vi "Framework Plugin Configuration Test.vi"() -> ()   [LabVIEW 2016]
uses:
  <vilib>/NI Veristand/VeriStand Data/Typedefs/Typedefs.Data Types.ctl
  Classes/Configuration.Transfer/Configuration.Transfer.lvclass
  Classes/Configuration.Channel/Configuration.Channel.lvclass
  Typedefs/Decimation Factors.ctl
  Classes/Plugin Model.UDP/Typedefs/UDP.Transfer Config.ctl
  Classes/Configuration.Transfer Group/Configuration.Transfer Group.lvclass
  Classes/Configuration.Channel/Configuration.Channel.lvclass/Configuration.Channel.ctl
  Classes/Configuration.Transfer/Configuration.Transfer.lvclass/Configuration.Transfer.ctl
  Classes/Configuration.Transfer Group/Configuration.Transfer Group.lvclass/Configuration.Transfer Group.ctl
  Classes/Plugin Model/Plugin Configuration.lvclass/Plugin Configuration.ctl
  Classes/Configuration.Channel/Properties/Write data type.vi
  Classes/Configuration.Channel/Properties/Write offset.vi
  Classes/Configuration.Transfer/Properties/Write byte order.vi
  Classes/Configuration.Transfer/Properties/Write decimation factors.vi
  Classes/Configuration.Transfer/Properties/Write Channels.vi
  Classes/Configuration.Transfer/Properties/Write custom config.vi
  Classes/Configuration.Transfer Group/Properties/Write Transfers.vi
  Classes/Plugin Model/Properties/Write Transfer Groups.vi
  Classes/Plugin Model.UDP/Plugin Configuration.UDP.lvclass
  C:/Users/Ryan/Documents/Git/Sourcetree/VeriStand-Data-Sharing-Framework/Source/Classes/Plugin Model/Plugin Configuration.lvclass
  <vilib>/NI Veristand/VeriStand Data/VeriStand Data.lvlib
  Classes/Plugin Model/Plugin Configuration.lvclass
panel:
  out "resource url":string
  out "Channels":cluster{"offset":u64, "data type":T1}[](array[cluster])
  out "required buffer size in bytes":u64
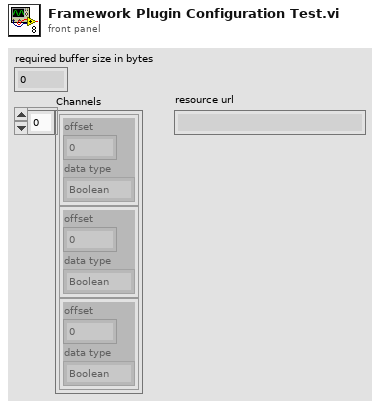
[diagram p1: front panel]
types:
  T1 = typedef "VeriStand Data.lvlib/Typedefs.Data Types.ctl" = enum16{"Boolean", "Single", "Double", "I8", "I16", "I32", "I64", "U8", "U16", "U32", "U64"}
  T2 = typedef "Plugin Configuration.UDP.lvclass/UDP.Transfer Config.ctl" = cluster{"port or service name":u16, "address":u32}
  T3 = typedef "Decimation Factors.ctl" = cluster{"decimation":u16, "offset":u16}
  T4 = enum16{"big-endian, network order", "native, host order", "little-endian"}
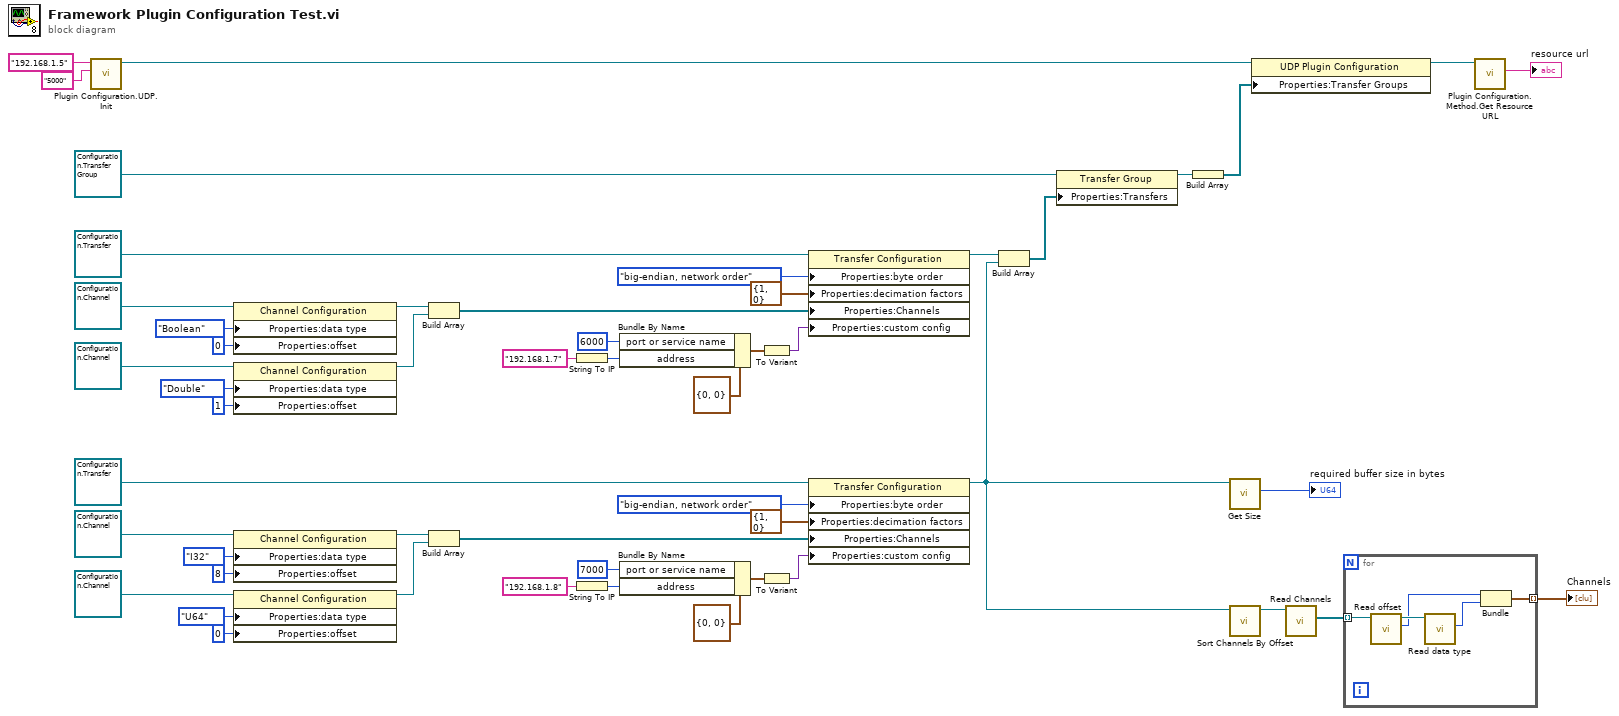
[diagram p0: block diagram]
diagram:
  n1 = call "Plugin Configuration.UDP.Init.vi"("Port"="5000", "IP Address"="192.168.1.5") -> ("UDP Plugin Configuration"=w1:refnum<class "Plugin Configuration.UDP.lvclass">)  [unwired: 8 in, 1 out]
  n2 = property class="Channel Configuration"(reference=refnum<class "Configuration.Channel.lvclass"> refnum ("Channel Configuration"), "Properties:data type"=Typedefs.Data_Types."Boolean" ("data type"), "Properties:offset"=u64 0 ("offset")) -> (reference out=w48:refnum<class "Configuration.Channel.lvclass">)  [unwired: 1 in, 1 out]
  n3 = property class="Channel Configuration"(reference=refnum<class "Configuration.Channel.lvclass"> refnum ("Channel Configuration"), "Properties:data type"=Typedefs.Data_Types."Double" ("data type"), "Properties:offset"=u64 1 ("offset")) -> (reference out=w47:refnum<class "Configuration.Channel.lvclass">)  [unwired: 1 in, 1 out]
  n4 = property class="Channel Configuration"(reference=refnum<class "Configuration.Channel.lvclass"> refnum ("Channel Configuration"), "Properties:data type"=Typedefs.Data_Types."I32" ("data type"), "Properties:offset"=u64 8 ("offset")) -> (reference out=w39:refnum<class "Configuration.Channel.lvclass">)  [unwired: 1 in, 1 out]
  n5 = property class="Channel Configuration"(reference=refnum<class "Configuration.Channel.lvclass"> refnum ("Channel Configuration"), "Properties:data type"=Typedefs.Data_Types."U64" ("data type"), "Properties:offset"=u64 0 ("offset")) -> (reference out=w38:refnum<class "Configuration.Channel.lvclass">)  [unwired: 1 in, 1 out]
  n6 = Build Array(w48, w47) -> (w46:refnum<class "Configuration.Channel.lvclass">[])
  n7 = Build Array(w39, w38) -> (w37:refnum<class "Configuration.Channel.lvclass">[])
  n8 = String To IP(1:"192.168.1.7" ("name")) -> (0:w13:u32)
  n9 = String To IP(1:"192.168.1.8" ("name")) -> (0:w8:u32)
  n10 = Bundle By Name(cluster=T2 {"port or service name"=0, "address"=0} ("UDP transfer config"), "port or service name"=u16 6000, "address"=w13) -> (w17:T2)
  n11 = Bundle By Name(cluster=T2 {"port or service name"=0, "address"=0} ("UDP transfer config"), "port or service name"=u16 7000, "address"=w8) -> (w11:T2)
  n12 = To Variant(anything=w17) -> (Variant=w16:variant)
  n13 = To Variant(anything=w11) -> (Variant=w7:variant)
  n14 = property class="Transfer Configuration"(reference=refnum<class "Configuration.Transfer.lvclass"> refnum ("Transfer Configuration"), "Properties:byte order"=T4."big-endian, network order" ("byte order"), "Properties:decimation factors"=T3 {"decimation"=1, "offset"=0} ("decimation factors"), "Properties:Channels"=w46, "Properties:custom config"=w16) -> (reference out=w34:refnum<class "Configuration.Transfer.lvclass">)  [unwired: 1 in, 1 out]
  n15 = property class="Transfer Configuration"(reference=refnum<class "Configuration.Transfer.lvclass"> refnum ("Transfer Configuration"), "Properties:byte order"=T4."big-endian, network order" ("byte order"), "Properties:decimation factors"=T3 {"decimation"=1, "offset"=0} ("decimation factors"), "Properties:Channels"=w37, "Properties:custom config"=w7) -> (reference out=w22:refnum<class "Configuration.Transfer.lvclass">)  [unwired: 1 in, 1 out]
  n16 = Build Array(w34, w22) -> (w5:refnum<class "Configuration.Transfer.lvclass">[])
  n17 = property class="Transfer Group"(reference=refnum<class "Configuration.Transfer Group.lvclass"> refnum ("Configuration.Transfer Group.lvclass"), "Properties:Transfers"=w5) -> (reference out=w3:refnum<class "Configuration.Transfer Group.lvclass">)  [unwired: 1 in, 1 out]
  n18 = Build Array(w3) -> (w2:refnum<class "Configuration.Transfer Group.lvclass">[])
  n19 = call "Get Size.vi"("Transfer Configuration in"=w22) -> ("size in bytes"=→"required buffer size in bytes":u64)  [unwired: 8 in, 2 out]
  n20 = call "Sort Channels By Offset.vi"("Transfer Configuration in"=w22) -> ("Transfer Configuration out"=w25:refnum<class "Configuration.Transfer.lvclass">)  [unwired: 9 in, 1 out]
  n21 = property class="UDP Plugin Configuration"(reference=w1, "Properties:Transfer Groups"=w2) -> (reference out=w20:refnum<class "Plugin Configuration.UDP.lvclass">)  [unwired: 1 in, 1 out]
  n22 = call "Read Channels.vi"("Configuration.Transfer in"=w25) -> ("Channels"=w24:refnum<class "Configuration.Channel.lvclass">[])  [unwired: 8 in, 2 out]
  n23 = for {
    tunnel: w24 -> [w56] mode=indexing
    tunnel: [w52] -> w23 mode=indexing
    n24 = call "Read offset.vi"("Configuration.Channel in"=w56) -> ("offset"=w54:u64, "Configuration.Channel out"=w55:refnum<class "Configuration.Channel.lvclass">)  [unwired: 8 in, 1 out]
    n25 = call "Read data type.vi"("Configuration.Channel in"=w55) -> ("data type"=w53:T1)  [unwired: 8 in, 2 out]
    n26 = Bundle("offset"=w54, "data type"=w53) -> (w52:cluster{"offset":u64, "data type":T1})  [unwired: 1 in]
  }
  "Channels" <- w23
  n27 = call "Plugin Configuration.Method.Get Resource URL.vi"("Plugin Model in"=w20) -> ("resource url"=→"resource url":string)  [unwired: 8 in, 2 out]
